vi "Range Auto Sacle Write.vi"(6 "Control Ref Queue":T1, 8 "error in (no error)":errorcluster, 9 "Range Auto Scale?":bool, 11 "3D Plot.lvclass in":refnum<class "3D Plot.lvclass">) -> (0 "error out":errorcluster, 3 "3D Plot.lvclass out":refnum<class "3D Plot.lvclass">)   [LabVIEW 2017, in "3D Plot.lvclass"]
uses:
  <vilib>/Math Plots/3D Math Plots/3D Plot/3D Plot/3D Plot.lvclass
  <vilib>/Math Plots/3D Math Plots/3D Plot/Action String/3DMathPlot Ctrl Act Queue.ctl
  <vilib>/Math Plots/3D Math Plots/3D Plot/Action String/3DMathPlot Ctrl Act Cluster.ctl
  <vilib>/Math Plots/3D Math Plots/3D Plot/Action String/3DMathPlot State Class.ctl
  <vilib>/Math Plots/3D Math Plots/3D Plot/3D Plot/3D Plot.lvclass/3D Plot.ctl
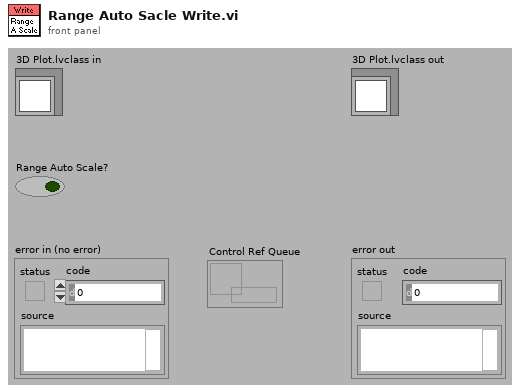
[diagram p1: front panel]
types:
  T1 = typedef "3DMathPlot Ctrl Act Queue.ctl" = refnum<queue>
  T2 = typedef "3D Plot.lvclass/Range Clusters.ctl" = cluster{"X Range":cluster{"Max X":sgl, "Min X":sgl}, "Y Range":cluster{"Max Y":sgl, "Min Y":sgl}, "Z Range":cluster{"Max Z":sgl, "Min Z":sgl}}
  T3 = cluster{"Auto Range X":bool, "Auto Range Y":bool, "Auto Range Z":bool}
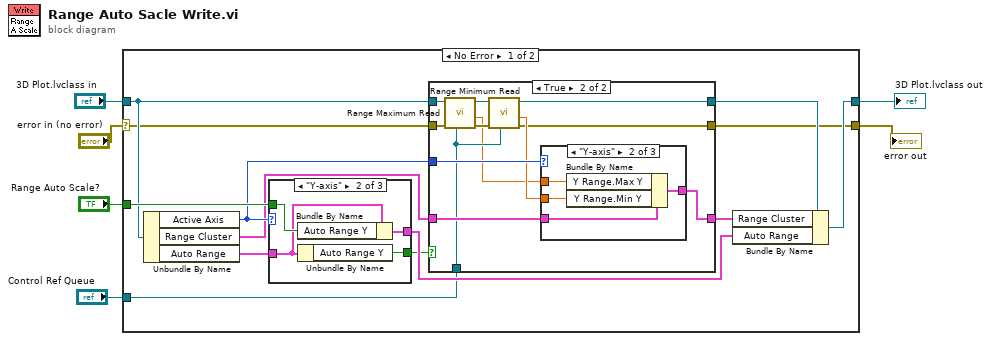
[diagram p0: block diagram]
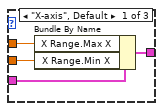
[diagram p3: hidden frame]
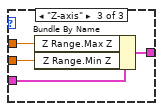
[diagram p4: hidden frame]
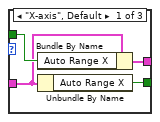
[diagram p5: hidden frame]
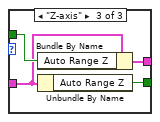
[diagram p6: hidden frame]
diagram:
  n1 = case shown="No Error" "error in (no error)" {
    selector: "error in (no error)" -> [w12 w59]
    tunnel: "Range Auto Scale?" -> [w19 _]
    tunnel: "3D Plot.lvclass in" -> [w14 w60]
    tunnel: [w17 w60] -> w4
    tunnel: [w11 w59] -> w2
    tunnel: "Control Ref Queue" -> [w16 _]
    frame No Error {
      n2 = Unbundle By Name(w14) -> ("Active Axis"=w10:enum16{"X-axis", "Y-axis", "Z-axis"}, "Range Cluster"=w8:T2, "Auto Range"=w9:T3)
      n3 = case shown="\"Y-axis\"" w10 {
        tunnel: w9 -> [w48 w52 w56]
        tunnel: w19 -> [w50 w54 w58]
        tunnel: [w49 w53 w57] -> w18
        tunnel: [w47 w51 w55] -> w15
        frame "X-axis", Default {
          n4 = Bundle By Name(cluster=w48, "Auto Range X"=w50) -> (w49:T3)
          n5 = Unbundle By Name(w48) -> ("Auto Range X"=w47:bool)
        }
        frame "Y-axis" {
          n6 = Bundle By Name(cluster=w52, "Auto Range Y"=w54) -> (w53:T3)
          n7 = Unbundle By Name(w52) -> ("Auto Range Y"=w51:bool)
        }
        frame "Z-axis" {
          n8 = Bundle By Name(cluster=w56, "Auto Range Z"=w58) -> (w57:T3)
          n9 = Unbundle By Name(w56) -> ("Auto Range Z"=w55:bool)
        }
      }
      n10 = case shown="True" w15 {
        tunnel: w14 -> [w22 w31]
        tunnel: [w22 w27] -> w13
        tunnel: w12 -> [w21 w30]
        tunnel: [w21 w25] -> w11
        tunnel: w10 -> [_ w34]
        tunnel: w8 -> [w20 w33]
        tunnel: [w20 w32] -> w7
        tunnel: w16 -> [_ w24]
        frame False {
        }
        frame True {
          n11 = call <vilib>:"Range Maximum Read.vi"("Control Ref Queue"=w24, "error in (no error)"=w30, "3D Plot.lvclass in"=w31) -> ("error out"=w26:errorcluster, "Range Max"=w23:sgl, "3D Plot.lvclass out"=w28:refnum<class "3D Plot.lvclass">)  [unwired: 6 out]
          n12 = call <vilib>:"Range Minimum Read.vi"("Control Ref Queue"=w24, "error in (no error)"=w26, "3D Plot.lvclass in"=w28) -> ("error out"=w25:errorcluster, "Range Min"=w29:sgl, "3D Plot.lvclass out"=w27:refnum<class "3D Plot.lvclass">)  [unwired: 6 out]
          n13 = case shown="\"Y-axis\"" w34 {
            tunnel: w33 -> [w38 w42 w46]
            tunnel: [w36 w41 w44] -> w32
            tunnel: w23 -> [w37 w40 w45]
            tunnel: w29 -> [w35 w39 w43]
            frame "X-axis", Default {
              n14 = Bundle By Name(cluster=w38, "X Range.Max X"=w37, "X Range.Min X"=w35) -> (w36:T2)
            }
            frame "Y-axis" {
              n15 = Bundle By Name(cluster=w42, "Y Range.Max Y"=w40, "Y Range.Min Y"=w39) -> (w41:T2)
            }
            frame "Z-axis" {
              n16 = Bundle By Name(cluster=w46, "Z Range.Max Z"=w45, "Z Range.Min Z"=w43) -> (w44:T2)
            }
          }
        }
      }
      n17 = Bundle By Name(cluster=w13, "Range Cluster"=w7, "Auto Range"=w18) -> (w17:refnum<class "3D Plot.lvclass">)
    }
    frame Error {
    }
  }
  "error out" <- w2
  "3D Plot.lvclass out" <- w4
